vi "Teleop.vi"(10 "Match Info":T1={"Autonomous Elapsed Seconds"=0.0, "TeleOp Elapsed Seconds"=0.0, "Disabled Elapsed Seconds"=0.0, "Visited Autonomous"=FALSE, "Visited TeleOp"=FALSE, "Visited Disabled"=FALSE, "Autonomous Settings"={"Autonomous Style"=enum."Independent", "VI Refnum"=refnum}}, 11 "Call Context":T2) -> ()   [LabVIEW 2012]
doc: "This VI is called for each TeleOp packet received from the DS where the robot is not disabled. It is often used to read from the joysticks and update I/O or to update setpoints for timed control loops. It should complete and return within 20 milliseconds or it may miss DS packets."
uses:
  <vilib>/Rock Robotics/WPI/DriverStation/WPI_DriverStationDerivedRobotMode.ctl
  <vilib>/Rock Robotics/WPI/DriverStation/WPI_DriverStationMatch Info.ctl
  Robot Global Data.vi
  <vilib>/Rock Robotics/WPI/Joystick/WPI_JoystickGetSetRefNum.vi
  <vilib>/Rock Robotics/WPI/Relay/WPI_RelayValue.ctl
panel:
  in  "PTO Disabled":dbl=90.0
  in  "PTO Enabled":dbl=140.0
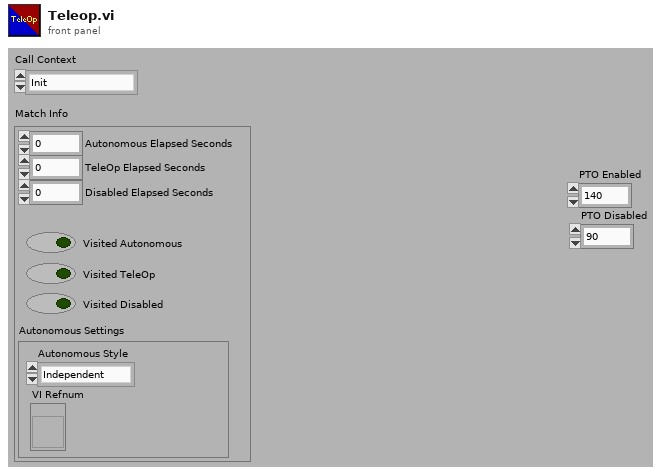
[diagram p1: front panel]
types:
  T1 = typedef "WPI_DriverStationMatch Info.ctl" = cluster{"Autonomous Elapsed Seconds":dbl, "TeleOp Elapsed Seconds":dbl, "Disabled Elapsed Seconds":dbl, "Visited Autonomous":bool, "Visited TeleOp":bool, "Visited Disabled":bool, "Autonomous Settings":cluster{"Autonomous Style":enum16{"Iterative", "Independent"}, "VI Refnum":refnum<vi>}}
  T2 = typedef "WPI_DriverStationDerivedRobotMode.ctl" = enum16{"Init", "Execute", "Stop"}
  T3 = typedef "WPI_MotorControlDeviceRef.ctl" = cluster{"DeviceStatus":errorcluster, "Type":enum16{"PWM", "CAN"}, "PWM":cluster{"Digital Module":T4, "PWM Channel":T5, "DeadBand":T6}, "CAN":cluster{"Device Number":u8, "Control Mode":T7, "Semaphore":T8, "Max Vout":dbl}, "Invert":bool, "TransformRef":T9, "InvTransformRef":T9}
  T4 = typedef "FPGA_TypedefDigitalModule.ctl" = enum16{"Digital Module 1", "Digital Module 2"}
  T5 = typedef "FPGA_DIOPWMChannel.ctl" = enum8{"PWM 1", "PWM 2", "PWM 3", "PWM 4", "PWM 5", "PWM 6", "PWM 7", "PWM 8", "PWM 9", "PWM 10", "Invalid"}
  T6 = typedef "WPI_PWMDeadband.ctl" = cluster{"Name":string, "maxPositivePwm":i32, "minPositivePwm":i32, "centerPwm":i32, "maxNegativePwm":i32, "minNegativePwm":i32, "angularRange":u16}
  T7 = typedef "WPI_CANJaguar_ControlMode.ctl" = enum8{"Percent VBus", "Current", "Speed", "Position", "Voltage"}
  T8 = typedef "Semaphore RefNum" = refnum<k1>
  T9 = typedef "WPI_PWMTransform_ConPane.ctl" = refnum<vi>
  T10 = cluster{"Driver Station Digital Input (1-8)[0]":bool, "Driver Station Digital Input (1-8)[1]":bool, "Driver Station Digital Input (1-8)[2]":bool, "Driver Station Digital Input (1-8)[3]":bool, "Driver Station Digital Input (1-8)[4]":bool, "Driver Station Digital Input (1-8)[5]":bool, "Driver Station Digital Input (1-8)[6]":bool, "Driver Station Digital Input (1-8)[7]":bool, "Driver Station Digital Input (1-8)[8]":bool}
  T11 = typedef "WPI_JoystickDevRef.ctl" = cluster{"Device":T12}
  T12 = typedef "WPI_JoystickDeviceEnum.ctl" = enum16{"USB 1", "USB 2", "USB 3", "USB 4", "Kinect 1", "Kinect 2"}
  T13 = cluster{"axis 1 (x)":dbl, "axis 2 (y)":dbl, "axis 3 (throttle)":dbl, "axis 4":dbl, "axis 5":dbl, "axis 6":dbl}
  T14 = typedef "WPI_ServoDeviceRef.ctl" = cluster{"DeviceStatus":errorcluster, "Digital Module":T4, "PWM Channel":T5, "DeadBand":T6}
  T15 = typedef "WPI_RelayValue.ctl" = enum16{"Off", "On", "Forward", "Reverse"}
  T16 = typedef "WPI_RelayDevRef.ctl" = cluster{"DevStatus":errorcluster, "Relay Channel":T17, "Digital Module":T4, "Relay Direction":T18}
  T17 = typedef "FPGA_DIORelayChannel.ctl" = enum8{"Relay 1", "Relay 2", "Relay 3", "Relay 4", "Relay 5", "Relay 6", "Relay 7", "Relay 8", "Invalid"}
  T18 = typedef "WPI_RelayDirection.ctl" = enum16{"Both directions", "Forward only", "Reverse only"}
  T19 = typedef "WPI_JoystickButtonState.ctl" = cluster{"Button 1":bool, "Button 2":bool, "Button 3":bool, "Button 4":bool, "Button 5":bool, "Button 6":bool, "Button 7":bool, "Button 8":bool, "Button 9":bool, "Button 10":bool, "Button 11":bool, "Button 12":bool}
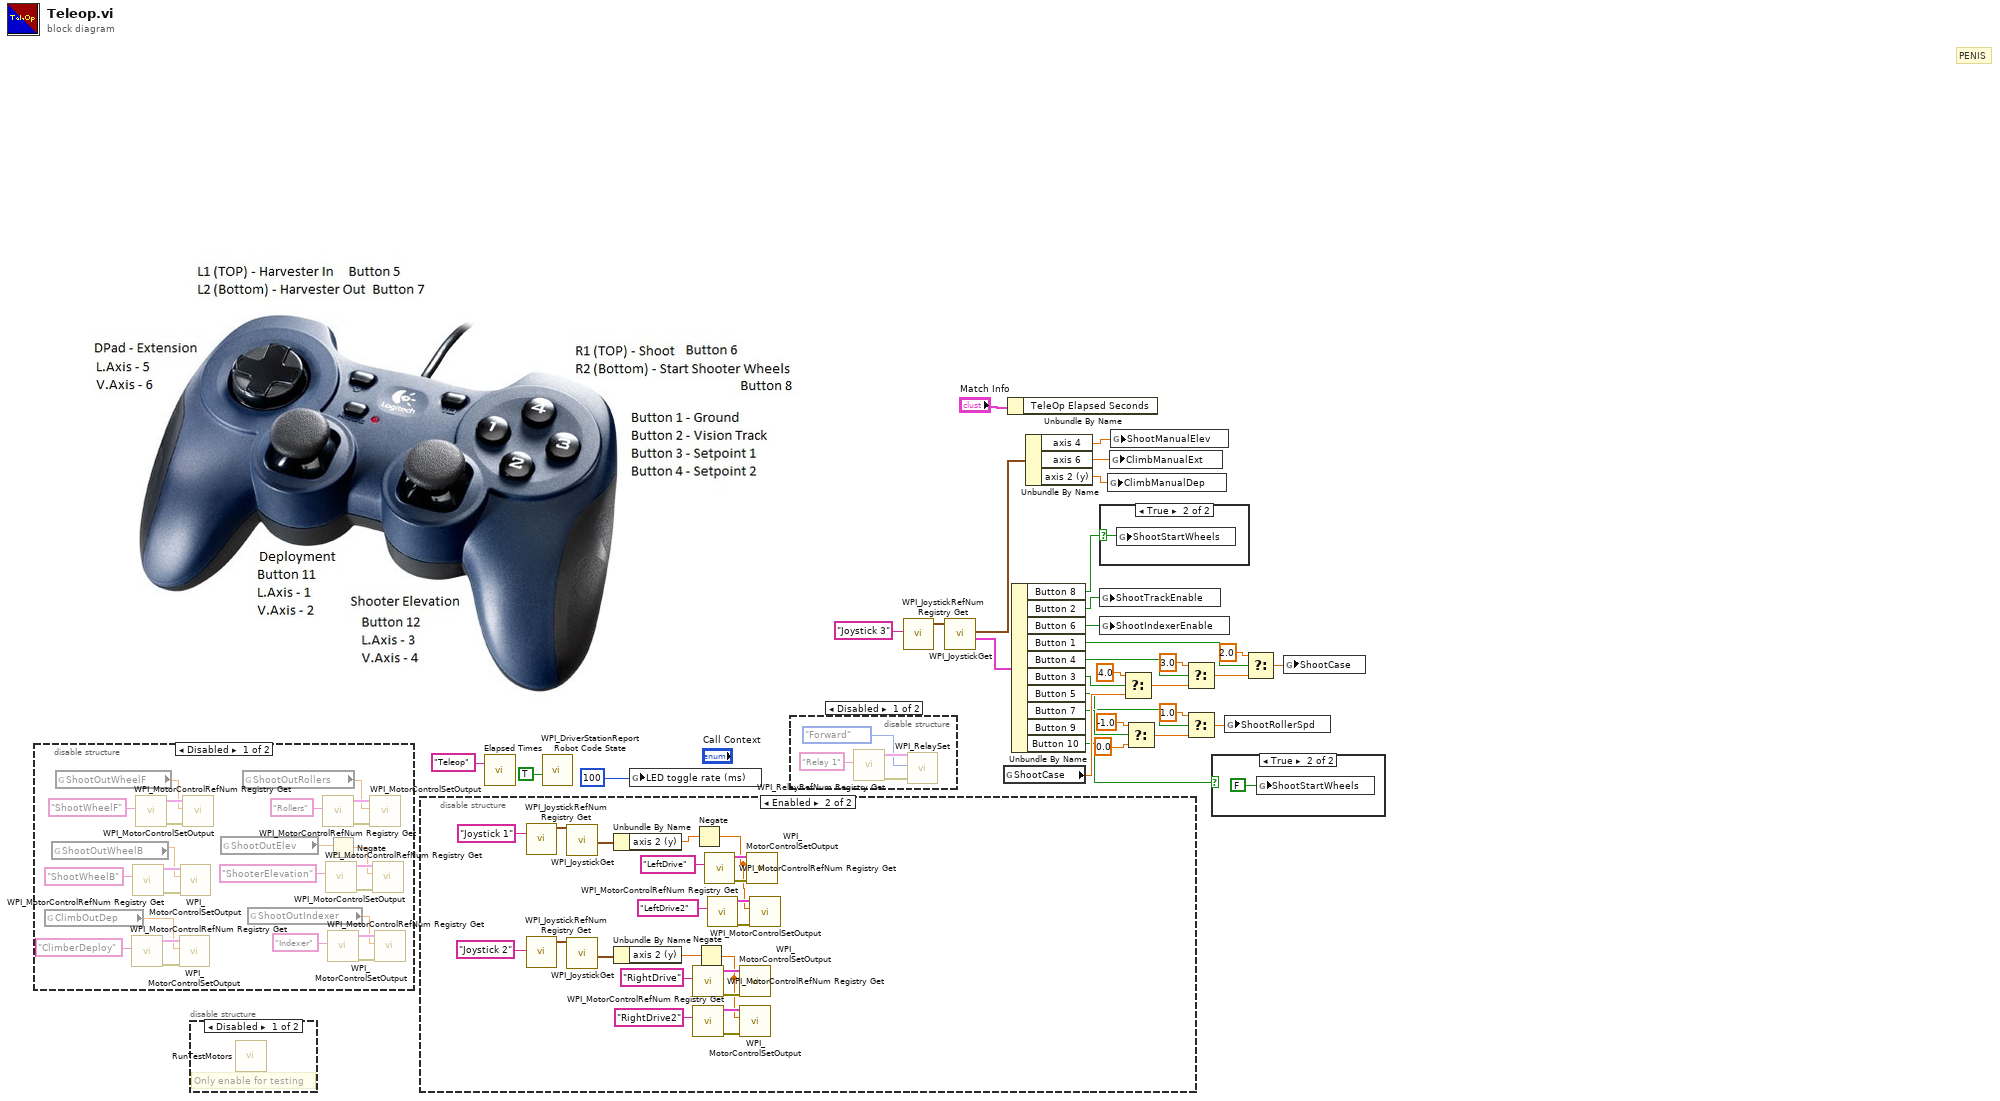
[diagram p0: block diagram]
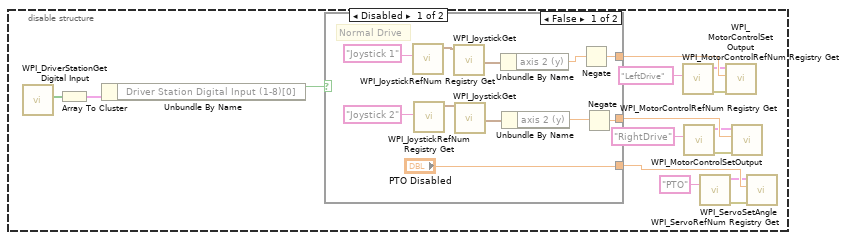
[diagram p4: hidden frame]
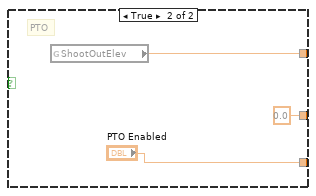
[diagram p5: hidden frame]
diagram:
  # "PENIS"
  n1 = disable-structure shown="Disabled" {
    frame Disabled {
      n2 = global read "Robot Global Data.vi" "ClimbOutDep"() -> (w33:dbl)
      n3 = global read "Robot Global Data.vi" "ShootOutWheelB"() -> (w34:dbl)
      n4 = global read "Robot Global Data.vi" "ShootOutWheelF"() -> (w39:dbl)
      n5 = call <vilib>:"WPI_MotorControlRefNum Registry Get.vi"("refnum name"="ClimberDeploy") -> ("error out"=w51:errorcluster, "MotorControlDevRef"=w50:T3)  [unwired: 9 in]
      n6 = call <vilib>:"WPI_MotorControlRefNum Registry Get.vi"("refnum name"="ShootWheelB") -> ("error out"=w52:errorcluster, "MotorControlDevRef"=w53:T3)  [unwired: 9 in]
      n7 = call <vilib>:"WPI_MotorControlRefNum Registry Get.vi"("refnum name"="ShootWheelF") -> ("error out"=w57:errorcluster, "MotorControlDevRef"=w56:T3)  [unwired: 9 in]
      n8 = call <vilib>:"WPI_MotorControlSetOutput.vi"("error in (no error)"=w51, "Output"=w33, "MotorControlDevRef"=w50) -> ()  [unwired: 6 in, 3 out]
      n9 = call <vilib>:"WPI_MotorControlSetOutput.vi"("error in (no error)"=w52, "Output"=w34, "MotorControlDevRef"=w53) -> ()  [unwired: 6 in, 3 out]
      n10 = call <vilib>:"WPI_MotorControlSetOutput.vi"("error in (no error)"=w57, "Output"=w39, "MotorControlDevRef"=w56) -> ()  [unwired: 6 in, 3 out]
      n11 = global read "Robot Global Data.vi" "ShootOutElev"() -> (w36:dbl)
      n12 = global read "Robot Global Data.vi" "ShootOutRollers"() -> (w37:dbl)
      n13 = global read "Robot Global Data.vi" "ShootOutIndexer"() -> (w38:dbl)
      n14 = call <vilib>:"WPI_MotorControlRefNum Registry Get.vi"("refnum name"="Rollers") -> ("error out"=w46:errorcluster, "MotorControlDevRef"=w47:T3)  [unwired: 9 in]
      n15 = call <vilib>:"WPI_MotorControlRefNum Registry Get.vi"("refnum name"="ShooterElevation") -> ("error out"=w45:errorcluster, "MotorControlDevRef"=w44:T3)  [unwired: 9 in]
      n16 = Negate(x=w36) -> (-x=w35:dbl)
      n17 = call <vilib>:"WPI_MotorControlRefNum Registry Get.vi"("refnum name"="Indexer") -> ("error out"=w40:errorcluster, "MotorControlDevRef"=w41:T3)  [unwired: 9 in]
      n18 = call <vilib>:"WPI_MotorControlSetOutput.vi"("error in (no error)"=w46, "Output"=w37, "MotorControlDevRef"=w47) -> ()  [unwired: 6 in, 3 out]
      n19 = call <vilib>:"WPI_MotorControlSetOutput.vi"("error in (no error)"=w45, "Output"=w35, "MotorControlDevRef"=w44) -> ()  [unwired: 6 in, 3 out]
      n20 = call <vilib>:"WPI_MotorControlSetOutput.vi"("error in (no error)"=w40, "Output"=w38, "MotorControlDevRef"=w41) -> ()  [unwired: 6 in, 3 out]
    }
    frame Enabled {
    }
  }
  n21 = disable-structure shown="Disabled" {
    frame Disabled {
      # "Only enable for testing"
      n22 = call "RunTestMotors.vi"() -> ()  [unwired: 16 in]
    }
    frame Enabled {
    }
  }
  n23 = disable-structure shown="Enabled" {
    frame Disabled {
      n24 = call <vilib>:"WPI_DriverStationGet Digital Input.vi"() -> ("Driver Station Digital Input (1-8)"=w72:bool[])  [unwired: 11 in]
      n25 = Array To Cluster(array=w72) -> (cluster=w71:T10)
      n26 = Unbundle By Name(w71) -> ("Driver Station Digital Input (1-8)[0]"=w70:bool)
      n27 = case shown="False" w70 {
        tunnel: [w75 w85] -> w67
        tunnel: [w74 0.0] -> w64
        tunnel: ["PTO Disabled" "PTO Enabled"] -> w61
        frame False {
          # "Normal Drive"
          n28 = call <vilib>:"WPI_JoystickRefNum Registry Get.vi"("refnum name"="Joystick 1") -> ("JoystickDevRef"=w77:T11)  [unwired: 1 in, 9 out]
          n29 = call <vilib>:"WPI_JoystickRefNum Registry Get.vi"("refnum name"="Joystick 2") -> ("JoystickDevRef"=w80:T11)  [unwired: 1 in, 9 out]
          n30 = call <vilib>:"WPI_JoystickGet.vi"("JoystickDevRef"=w77) -> ("Axes"=w78:T13)  [unwired: 1 in, 5 out]
          n31 = call <vilib>:"WPI_JoystickGet.vi"("JoystickDevRef"=w80) -> ("Axes"=w79:T13)  [unwired: 1 in, 5 out]
          n32 = Unbundle By Name(w78) -> ("axis 2 (y)"=w83:dbl)
          n33 = Unbundle By Name(w79) -> ("axis 2 (y)"=w82:dbl)
          n34 = Negate(x=w83) -> (-x=w75:dbl)
          n35 = Negate(x=w82) -> (-x=w74:dbl)
        }
        frame True {
          # "PTO"
          n36 = global read "Robot Global Data.vi" "ShootOutElev"() -> (w85:dbl)
        }
      }
      n37 = call <vilib>:"WPI_MotorControlRefNum Registry Get.vi"("refnum name"="LeftDrive") -> ("error out"=w65:errorcluster, "MotorControlDevRef"=w66:T3)  [unwired: 9 in]
      n38 = call <vilib>:"WPI_MotorControlRefNum Registry Get.vi"("refnum name"="RightDrive") -> ("error out"=w62:errorcluster, "MotorControlDevRef"=w63:T3)  [unwired: 9 in]
      n39 = call <vilib>:"WPI_ServoRefNum Registry Get.vi"("refnum name"="PTO") -> ("error out"=w60:errorcluster, "ServoDeviceRef"=w59:T14)  [unwired: 9 in]
      n40 = call <vilib>:"WPI_MotorControlSetOutput.vi"("error in (no error)"=w65, "Output"=w67, "MotorControlDevRef"=w66) -> ()  [unwired: 6 in, 3 out]
      n41 = call <vilib>:"WPI_MotorControlSetOutput.vi"("error in (no error)"=w62, "Output"=w64, "MotorControlDevRef"=w63) -> ()  [unwired: 6 in, 3 out]
      n42 = call <vilib>:"WPI_ServoSetAngle.vi"("error in (no error)"=w60, "Angle"=w61, "ServoDeviceRef"=w59) -> ()  [unwired: 7 in, 2 out]
    }
    frame Enabled {
      n43 = call <vilib>:"WPI_JoystickRefNum Registry Get.vi"("refnum name"="Joystick 1") -> ("JoystickDevRef"=w101:T11)  [unwired: 1 in, 9 out]
      n44 = call <vilib>:"WPI_JoystickRefNum Registry Get.vi"("refnum name"="Joystick 2") -> ("JoystickDevRef"=w103:T11)  [unwired: 1 in, 9 out]
      n45 = call <vilib>:"WPI_JoystickGet.vi"("JoystickDevRef"=w101) -> ("Axes"=w96:T13)  [unwired: 1 in, 5 out]
      n46 = call <vilib>:"WPI_JoystickGet.vi"("JoystickDevRef"=w103) -> ("Axes"=w102:T13)  [unwired: 1 in, 5 out]
      n47 = Unbundle By Name(w96) -> ("axis 2 (y)"=w97:dbl)
      n48 = Unbundle By Name(w102) -> ("axis 2 (y)"=w105:dbl)
      n49 = call <vilib>:"WPI_MotorControlRefNum Registry Get.vi"("refnum name"="RightDrive") -> ("error out"=w106:errorcluster, "MotorControlDevRef"=w108:T3)  [unwired: 9 in]
      n50 = call <vilib>:"WPI_MotorControlRefNum Registry Get.vi"("refnum name"="RightDrive2") -> ("error out"=w90:errorcluster, "MotorControlDevRef"=w88:T3)  [unwired: 9 in]
      n51 = Negate(x=w97) -> (-x=w91:dbl)
      n52 = Negate(x=w105) -> (-x=w87:dbl)
      n53 = call <vilib>:"WPI_MotorControlRefNum Registry Get.vi"("refnum name"="LeftDrive") -> ("error out"=w93:errorcluster, "MotorControlDevRef"=w98:T3)  [unwired: 9 in]
      n54 = call <vilib>:"WPI_MotorControlRefNum Registry Get.vi"("refnum name"="LeftDrive2") -> ("error out"=w92:errorcluster, "MotorControlDevRef"=w94:T3)  [unwired: 9 in]
      n55 = call <vilib>:"WPI_MotorControlSetOutput.vi"("error in (no error)"=w106, "Output"=w87, "MotorControlDevRef"=w108) -> ()  [unwired: 6 in, 3 out]
      n56 = call <vilib>:"WPI_MotorControlSetOutput.vi"("error in (no error)"=w90, "Output"=w87, "MotorControlDevRef"=w88) -> ()  [unwired: 6 in, 3 out]
      n57 = call <vilib>:"WPI_MotorControlSetOutput.vi"("error in (no error)"=w93, "Output"=w91, "MotorControlDevRef"=w98) -> ()  [unwired: 6 in, 3 out]
      n58 = call <vilib>:"WPI_MotorControlSetOutput.vi"("error in (no error)"=w92, "Output"=w91, "MotorControlDevRef"=w94) -> ()  [unwired: 6 in, 3 out]
    }
  }
  n59 = call "Elapsed Times.vi"("Call Name"="Teleop") -> ()  [unwired: 2 in, 1 out]
  n60 = call <vilib>:"WPI_DriverStationReport Robot Code State.vi"("TeleOp"=TRUE ("Autonomous")) -> ()  [unwired: 10 in, 1 out]
  n61 = global write "Robot Global Data.vi" "LED toggle rate (ms)"(u32 100 ("LED ms toggle rate")) -> ()
  n62 = disable-structure shown="Disabled" {
    frame Disabled {
      n63 = call <vilib>:"WPI_RelayRefNum Registry Get.vi"("refnum name"="Relay 1") -> ("error out"=w110:errorcluster, "RelayDevRef"=w112:T16)  [unwired: 9 in]
      n64 = call <vilib>:"WPI_RelaySet.vi"("error in (no error)"=w110, "RelayValue"=WPI_RelayValue."Forward", "RelayDevRef"=w112) -> ()  [unwired: 7 in, 2 out]
    }
    frame Enabled {
    }
  }
  n65 = call <vilib>:"WPI_JoystickRefNum Registry Get.vi"("refnum name"="Joystick 3") -> ("JoystickDevRef"=w29:T11)  [unwired: 9 in, 1 out]
  n66 = call <vilib>:"WPI_JoystickGet.vi"("JoystickDevRef"=w29) -> ("Buttons"=w27:T19, "Axes"=w26:T13)  [unwired: 4 in, 1 out]
  n67 = global read "Robot Global Data.vi" "ShootCase"() -> (w13:dbl)
  n68 = Unbundle By Name("Match Info") -> ()  [unwired: 1 out]
  n69 = Unbundle By Name(w27) -> ("Button 8"=w4:bool, "Button 2"=w24:bool, "Button 6"=w25:bool, "Button 1"=w21:bool, "Button 4"=w19:bool, "Button 3"=w18:bool, "Button 5"=w9:bool, "Button 7"=w11:bool, "Button 10"=w3:bool)  [unwired: 1 out]
  n70 = Unbundle By Name(w26) -> ("axis 4"=w23:dbl, "axis 6"=w22:dbl, "axis 2 (y)"=w2:dbl)
  n71 = case shown="True" w4 {
    selector: w4 -> [_ w113]
    frame False {
    }
    frame True {
      n72 = global write "Robot Global Data.vi" "ShootStartWheels"(w113) -> ()
    }
  }
  n73 = global write "Robot Global Data.vi" "ShootTrackEnable"(w24) -> ()
  n74 = global write "Robot Global Data.vi" "ShootIndexerEnable"(w25) -> ()
  n75 = global write "Robot Global Data.vi" "ClimbManualDep"(w2) -> ()
  n76 = global write "Robot Global Data.vi" "ClimbManualExt"(w22) -> ()
  n77 = global write "Robot Global Data.vi" "ShootManualElev"(w23) -> ()
  n78 = Select(t=4.0, s=w18, f=w13) -> (s? t:f=w17:dbl)
  n79 = Select(t=-1.0, s=w11, f=0.0) -> (s? t:f=w10:dbl)
  n80 = Select(t=3.0, s=w19, f=w17) -> (s? t:f=w15:dbl)
  n81 = Select(t=1.0, s=w9, f=w10) -> (s? t:f=w5:dbl)
  n82 = case shown="True" w3 {
    frame False {
    }
    frame True {
      n83 = global write "Robot Global Data.vi" "ShootStartWheels"(FALSE ("ShootStartWheels")) -> ()
    }
  }
  n84 = global write "Robot Global Data.vi" "ShootRollerSpd"(w5) -> ()
  n85 = Select(t=2.0, s=w21, f=w15) -> (s? t:f=w12:dbl)
  n86 = global write "Robot Global Data.vi" "ShootCase"(w12) -> ()
